vi "OneSessOnePinOneInstrOneSiteReservation_CallGetConnectionFromPinForNonExistentPin_ReturnsError.vi"(8 "error in":errorcluster) -> (0 "error out":errorcluster, 2 "result":string, 3 "pass":bool)   [LabVIEW 2020, in "MeasurementServerTests.lvlib"]
uses:
  MeasurementServerTests.lvlib
  Runtime/MeasurementLink Session Management/Session Reservation/Connection.ctl
  Runtime/MeasurementLink Session Management/Session Reservation/Hardware Independent Connection.ctl
  8c161b2c-7580-4f71-9eec-17cc94e5f6f8.vi
  8c161b2c-7580-4f71-9eec-17cc94e5f6f8.vi/d089b476-b30c-4b91-b2ff-fbae0086b065.vi
  Runtime/MeasurementLink Session Management/Session Reservation/Get Connections Impl.vi
  Runtime/MeasurementLink Measurement Server/Helpers/Error Strings Global Internal.vi
  <vilib>/Utility/error.llb/Error Cluster From Error Code.vi
  Runtime/MeasurementLink Session Management/Session Reservation/Session Reservation.lvclass
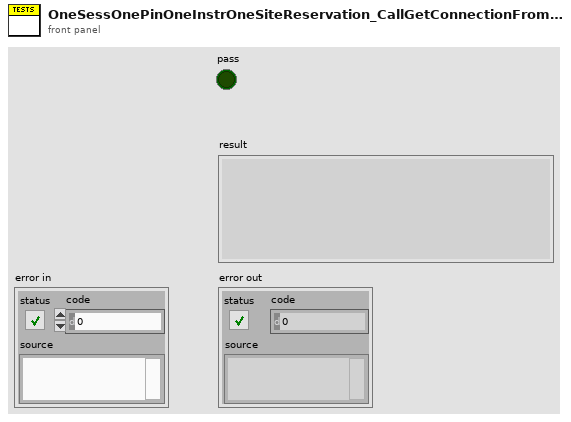
[diagram p1: front panel]
types:
  T1 = typedef "MeasurementLink Session Management.lvlib/Session Reservation.lvclass/Connection.ctl" = cluster{"connection":T2, "session":variant}
  T2 = typedef "MeasurementLink Session Management.lvlib/Session Reservation.lvclass/Hardware Independent Connection.ctl" = cluster{"pin or relay name":string, "site":i32, "instrument type id":string, "channel":string}
  T3 = typedef "MeasurementLink Session Management.lvlib/Session Reservation.lvclass/Data.ctl" = cluster{"session and driver infos":T4[], "pins":string[]}
  T4 = typedef "MeasurementLink Session Management.lvlib/Session Reservation.lvclass/Session and Driver Info.ctl" = cluster{"session info":T5, "session created":bool, "session":variant}
  T5 = typedef "MeasurementLink Session Management Client.lvlib/ni_measurementlink_sessionmanagement_v1_SessionInformation.ctl" = cluster{"session":T6, "resource_name":string, "channel_list":string, "instrument_type_id":string, "session_exists":bool, "channel_mappings":T7[]}
  T6 = typedef "MeasurementLink Session Management Client.lvlib/nidevice_grpc_Session.ctl" = cluster{"name":string}
  T7 = typedef "MeasurementLink Session Management Client.lvlib/ni_measurementlink_sessionmanagement_v1_ChannelMapping.ctl" = cluster{"pin_or_relay_name":string, "site":i32, "channel":string}
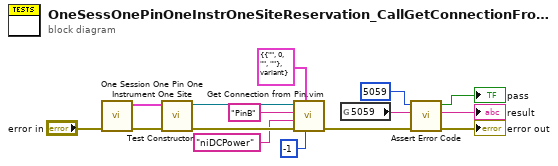
[diagram p0: block diagram]
diagram:
  n1 = call "One Session One Pin One Instrument One Site.vi"("error in"="error in") -> ("error out"=w3:errorcluster, "data out"=w2:T3)  [unwired: 9 in]
  n2 = call "Test Constructor.vi"("error in"=w3, "data"=w2) -> ("error out"=w14:errorcluster, "Session Reservation out"=w13:refnum<class "Session Reservation.lvclass">)  [unwired: 8 in]
  n3 = call "Get Connection from Pin.vim"("site"=-1, "connection type"=T1 {"connection"={"pin or relay name"="", "site"=0, "instrument type id"="", "channel"=""}, "session"=variant} ("connection"), "error in"=w14, "instrument type id"="niDCPower", "pin or relay name"="PinB", "session reservation in"=w13) -> ("error out"=w7:errorcluster)  [unwired: 3 in, 2 out]
  n4 = global read "Error Strings Global Internal.vi" "5059"() -> (w5:string)
  n5 = call "Assert Error Code.vi"("error in"=w7, "expected error description"=w5, "expected error code"=5059) -> ("error out"=→"error out":errorcluster, "details"=→"result":string, "error code match?"=→"pass":bool)  [unwired: 6 in]
